vi "Scan_Continuous.vi"(3 "Error In":errorcluster, 5 "Cluster Count":dbl=1.0) -> (0 "Error Out":errorcluster, 2 "XY Graph":cluster{"X":dbl, "Y":dbl}[](graph))   [LabVIEW 2016, in "Hokuyo_URG.lvlib"]
uses:
  Hokuyo_URG.lvlib
  <instrlib>/Hokuyo URG Series/Public/Initialize-Standard.vi
  <instrlib>/Hokuyo URG Series/Hokuyo URG Series.lvlib
panel:
  in  "stop":bool
  in  "VISA resource name":refnum<visa-resource-name>="COM3"
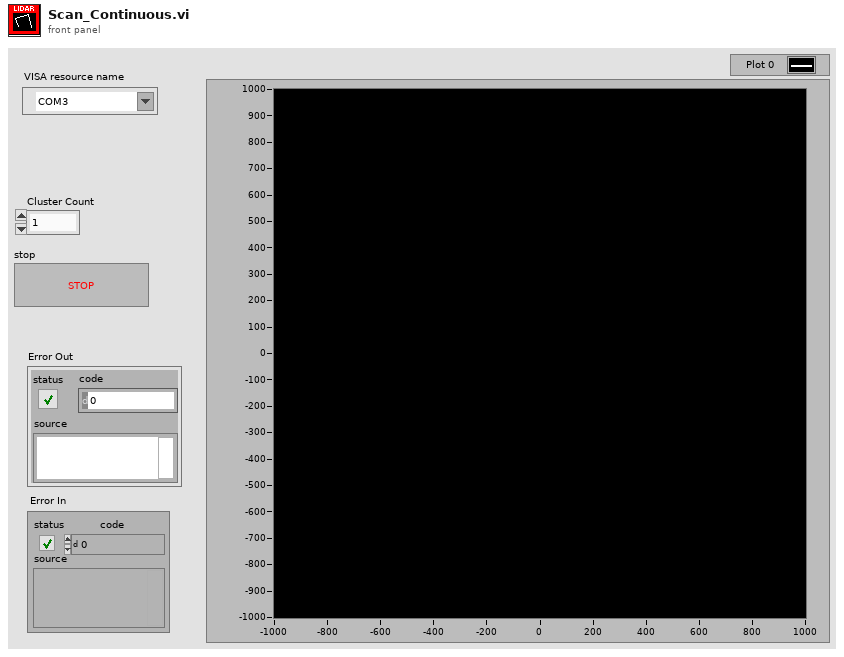
[diagram p1: front panel]
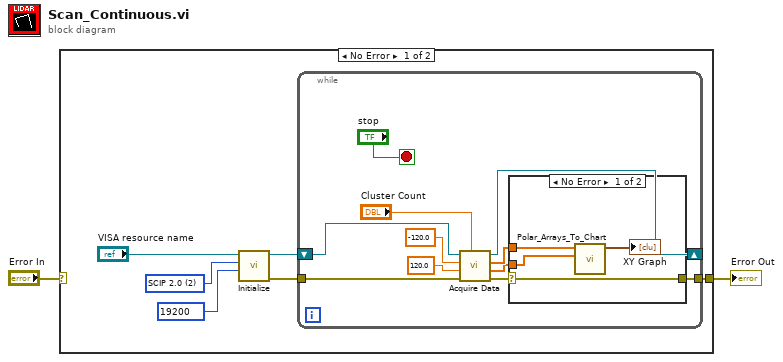
[diagram p0: block diagram]
diagram:
  n1 = case shown="No Error" "Error In" {
    selector: "Error In" -> [_ w25]
    tunnel: [w3 w25] -> w2
    frame No Error {
      w6 = u32 19200 items=["19200"=19200, "57600"=57600, "115200"=115200, "250000"=250000, "500000"=500000, "750000"=750000] ("Serial Configuration (19200 : 19200 Baud)")
      w7 = u32 2 items=["Convert to Latest", "SCIP 1.1", "SCIP 2.0"] ("Protocol (2: SCIP 2.0)")
      n2 = call-poly <instrlib>:"Initialize.vi"("Serial Configuration (19200 : 19200 Baud)"=w6, "Protocol (2: SCIP 2.0)"=w7, "VISA resource name"="VISA resource name") -> ("error out"=w4:errorcluster, "VISA resource name out"=w5:refnum<visa-resource-name>)  [unwired: 7 in]
      n3 = while {
        tunnel: w4 -> [w18]
        shift-right: [w14] -> _
        shift-left: w5 -> [w19]
        tunnel: [w10] -> w3
        stop <- "stop" stop-if-true
        n4 = call <instrlib>:"Acquire Data.vi"("Cluster Count (1)"="Cluster Count", "error in (no error)"=w18, "End Point (120°)"=120.0, "Start Point (-120°)"=-120.0, "VISA resource name"=w19) -> ("error out"=w15:errorcluster, "Direction"=w12:dbl[], "Magnitude"=w13:dbl[], "VISA resource name out"=w14:refnum<visa-resource-name>)  [unwired: 3 in]
        n5 = case shown="No Error" w15 {
          selector: w15 -> [w21 w24]
          tunnel: w13 -> [w23 _]
          tunnel: w12 -> [w22 _]
          tunnel: [w21 w24] -> w10
          frame No Error {
            n6 = call "Polar_Arrays_To_Chart.vi"("Direction"=w22, "Magnitude"=w23) -> ("Scan"=→"XY Graph":cluster{"x":dbl, "y":dbl}[])  [unwired: 9 in]
          }
          frame Error {
          }
        }
      }
    }
    frame Error {
    }
  }
  "Error Out" <- w2
